vi "SR_Gen_Overview.vi"(11 "State Sample":refnum<class "RDS State.lvclass">) -> (2 "Overview":T1 {"Distance to Target" format="%.01f [meters]"; "Longitude" format="%.6g"; "Latitude" format="%.6g"; "Water Temp" format="%.0f [celcius]"; "Pitch" scale=45.0..-45.0; "Roll" scale=-20.0..20.0; "Current" format="%02.2f [amps]"; "Voltage" format="%02.2f [volts]"; "Capacity" format="%_1f [Percent]"; "Water Depth" format="%.01f [meters]"; "GPS Speed" format="%.01f [knots]"; "Compass" scale=0.36..360.0}, 3 "State Sample Out":refnum<class "RDS State.lvclass">)   [LabVIEW 2015, in "Shore Library.lvlib"]
uses:
  Shore Library.lvlib
  SR_Overview.ctl
  RDS State Tracker/RDS State/RDS State.lvclass
  RDS State Tracker/RDS State/RDS State.lvclass/RDS State.ctl
panel:
  # "Batteries"
  # "Actual Heading"
  # "Desired Heading"
  # "Throttle"
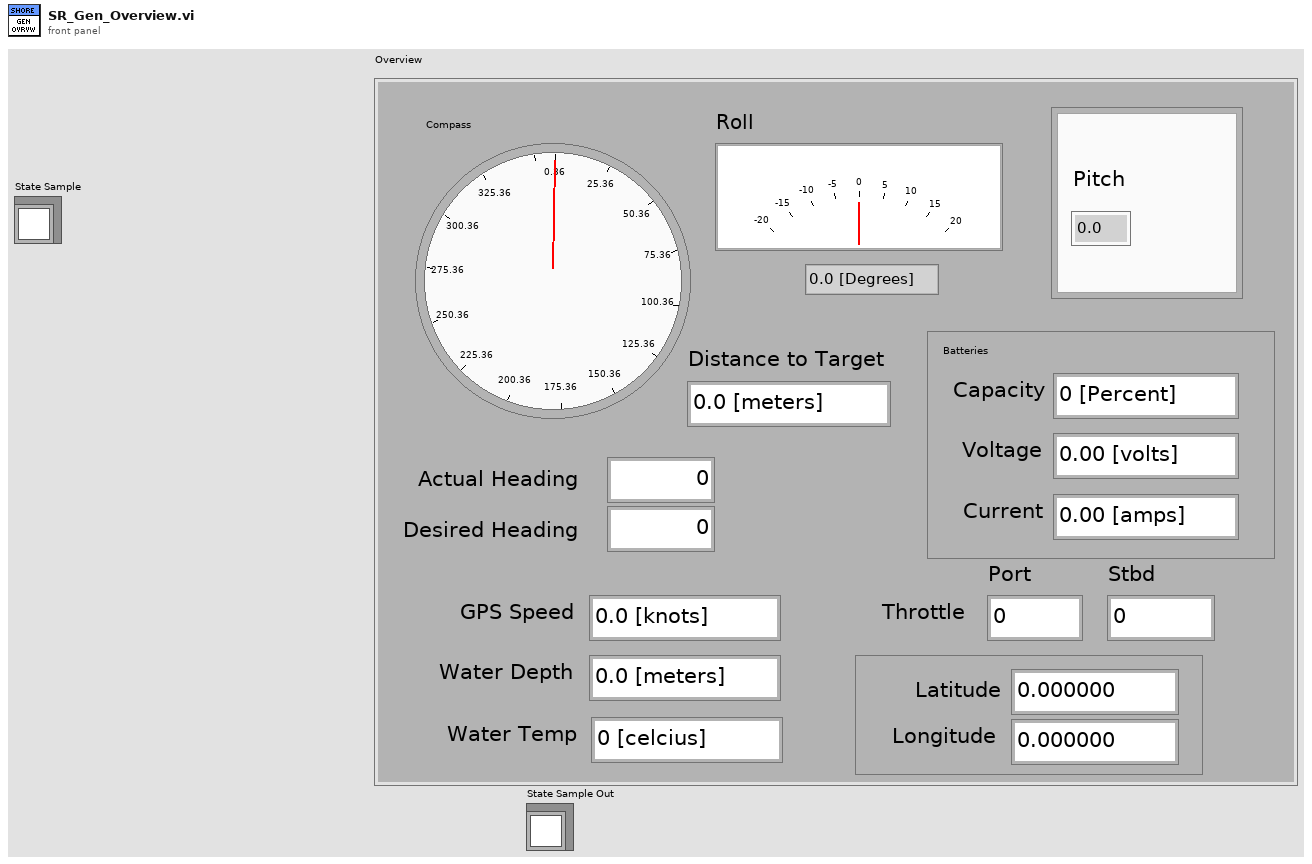
[diagram p1: front panel]
types:
  T1 = typedef "Shore Library.lvlib/SR_Overview.ctl" = cluster{"Throttle Stbd":dbl, "Compass":cluster{sgl, sgl}, "GPS Speed":dbl, "Water Depth":dbl, "Capacity":dbl, "Voltage":dbl, "Current":dbl, "Throttle Port":dbl, "Roll":sgl, "Pitch":sgl, "Water Temp":dbl, "Latitude":dbl, "Longitude":dbl, "Distance to Target":dbl}
  T2 = typedef "RDS Instrument Library.lvlib/Battery Data.ctl" = cluster{"Battery Status":T3, "Pack Voltage":sgl, "Pack Current":sgl, "Pack Capacity":sgl, "Max Cell Temp":sgl, "Min Cell Temp":sgl, "Max Cell Voltage":sgl, "Min Cell Voltage":sgl}
  T3 = typedef "RDS Instrument Library.lvlib/Battery Status.ctl" = enum16{"Pack Normal", "Alarm: Cell temp too high", "Alarm: Pack voltage too high", "Warn: Pack voltage too high ", "Alarm: Pack voltage too low", "Warn: Pack voltage low", "Alarm Pack current too high", "Warn: Pack current too high ", "Fault: Pack to chassis connection detected", "Fault: Pack to cell connection error", "Fautl: System error"}
  T4 = typedef "RDS Child Messages.lvlib/Depth Data.ctl" = cluster{"Depth":sgl, "Water Temp":i8}
  T5 = typedef "RDS Child Messages.lvlib/Helm Status Control.ctl" = cluster{"Helm State":T6, "Heading Command Control":T7, "Steering Command Control":T8, "Last Command Time":timestamp, "Gains":T9, "Current Heading":dbl, "Port Throttle":i16, "STBD Throttle":i16, "Limiter":dbl}
  T6 = typedef "RDS Helm Actor.lvlib/Helm State.ctl" = enum16{"Idle", "Executing Heading Command", "Executing Steering Command"}
  T7 = typedef "RDS Child Messages.lvlib/Heading Command Cntrl.ctl" = cluster{"Throttle":i16, "Heading":sgl, "Duration (s)":i16}
  T8 = typedef "RDS Child Messages.lvlib/Steering Command Cntrl.ctl" = cluster{"Throttle":i16, "Rudder":i8, "Duration (s)":u16}
  T9 = typedef "RDS Child Messages.lvlib/PID Gains Control.ctl" = cluster{"P (Kc)":sgl, "I (Ti)":sgl, "D (Td)":sgl}
  T10 = typedef "RDS Child Messages.lvlib/MCB Motor Status.ctl" = cluster{"Motor Power":i16, "Motor Command":i16, "Battery Volts":sgl, "Battery Amps":sgl, "Motor Amps":sgl, "MCU Temp":i16, "Heatsink Temp":i16, "Fault Flags":u16, "StatusFlags":u16}
  T11 = typedef "RDS Instrument Library.lvlib/Compass Data.ctl" = cluster{"Compass Heading":sgl, "pitch Angle":sgl, "roll Angle":sgl, "Temperature":sgl, "Depth":sgl, "Magnetic Field":sgl, "Magnetic Field X":sgl, "Magnetic Field Y":sgl, "Magnetic Field Z":sgl, "Acceleration":sgl, "Acceleration X":sgl, "Acceleration Y":sgl, "Gyro":sgl, "Gyro X":sgl, "Acceleration Z":sgl, "Gyro Y":sgl, "Raw Heading":sgl}
  T12 = typedef "RDS Libraries.lvlib/NMEA.lvlib/NMEA_GPRMC-data.ctl" = cluster{"TimeStamp":timestamp, "Validity":bool, "Latitude":dbl, "Latitude-Direction":T13, "Longitude":dbl, "Longitude-Direction":T14, "Speed in knots":sgl, "True course":sgl, "Date Stamp":timestamp, "Magnetic Variation (East/West)":sgl, "GPS Latitude":dbl, "GPS Longitude":dbl}
  T13 = typedef "RDS Libraries.lvlib/NMEA.lvlib/NMEA_LatitudeDirection.ctl" = enum16{"", "North", "South"}
  T14 = typedef "RDS Libraries.lvlib/NMEA.lvlib/NMEA_LongitudeDirection.ctl" = enum16{"", "East", "West"}
  T15 = typedef "RDS Child Messages.lvlib/Mission Controller State Message.lvclass/Mission Controller State Control.ctl" = cluster{"iHasControl":bool, "controlTimer":timestamp, "Nav State":T16, "Current MissionOp Index":i32, "Mission":T17[], "Distance to Target":dbl, "Seconds to Timeout":dbl}
  T16 = typedef "RDS Mission Controller Actor.lvlib/Mission Controller Navigation State.ctl" = cluster{"GPS Latitude":ext, "GPS Longitude":ext, "Compass Heading":dbl, "Speed":dbl}
  T17 = typedef "RDS Mission Controller Actor.lvlib/MissionOp.ctl" = cluster{"MissionOp Type":enum16{"Waypoint", "Loiter", "Wait", "Deploy AIP", "Stow AIP"}, "Duration (s)":u16, "Throttle":i16, "GPS Latitude":dbl, "GPS Longitude":dbl, "Loiter Range (m)":u16}
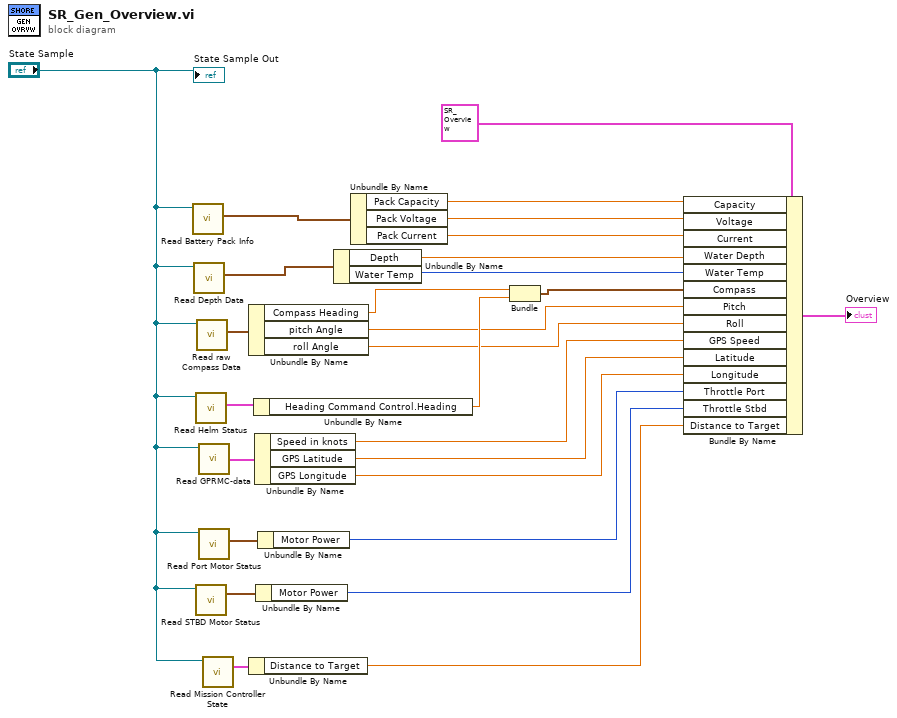
[diagram p0: block diagram]
diagram:
  n1 = call "Read Battery Pack Info.vi"("RDS State in"="State Sample") -> ("Battery Pack Info"=w27:T2)  [unwired: 8 in, 2 out]
  n2 = call "Read Depth Data.vi"("RDS State in"="State Sample") -> ("Depth Data"=w22:T4)  [unwired: 8 in, 2 out]
  n3 = call "Read Helm Status.vi"("RDS State in"="State Sample") -> ("Helm Status"=w19:T5)  [unwired: 8 in, 2 out]
  n4 = call "Read STBD Motor Status.vi"("RDS State in"="State Sample") -> ("STBD Motor"=w6:T10)  [unwired: 8 in, 2 out]
  n5 = call "Read raw Compass Data.vi"("RDS State in"="State Sample") -> ("Compass Data"=w18:T11)  [unwired: 8 in, 2 out]
  n6 = call "Read GPRMC-data.vi"("RDS State in"="State Sample") -> ("GPRMC-data"=w12:T12)  [unwired: 8 in, 2 out]
  n7 = call "Read Port Motor Status.vi"("RDS State in"="State Sample") -> ("Port Motor Data"=w8:T10)  [unwired: 8 in, 2 out]
  n8 = call "Read Mission Controller State.vi"("RDS State in"="State Sample") -> ("Mission Controller State"=w3:T15)  [unwired: 8 in, 2 out]
  n9 = Unbundle By Name(w18) -> ("Compass Heading"=w17:sgl, "pitch Angle"=w14:sgl, "roll Angle"=w13:sgl)
  n10 = Unbundle By Name(w3) -> ("Distance to Target"=w1:dbl)
  n11 = Unbundle By Name(w19) -> ("Heading Command Control.Heading"=w16:sgl)
  n12 = Unbundle By Name(w12) -> ("Speed in knots"=w11:sgl, "GPS Latitude"=w10:dbl, "GPS Longitude"=w9:dbl)
  n13 = Unbundle By Name(w6) -> ("Motor Power"=w5:i16)
  n14 = Unbundle By Name(w8) -> ("Motor Power"=w7:i16)
  n15 = Unbundle By Name(w22) -> ("Depth"=w21:sgl, "Water Temp"=w20:i8)
  n16 = Unbundle By Name(w27) -> ("Pack Capacity"=w26:sgl, "Pack Voltage"=w25:sgl, "Pack Current"=w24:sgl)
  n17 = Bundle("Compass Heading"=w17, "Heading"=w16) -> (w15:cluster{"Compass Heading":sgl, "Heading":sgl})  [unwired: 1 in]
  n18 = Bundle By Name(cluster=T1 {"Throttle Stbd"=0.0, "Compass"={7.9180083, 358.98358}, "GPS Speed"=0.0, "Water Depth"=0.0, "Capacity"=0.0, "Voltage"=0.0, "Current"=0.0, "Throttle Port"=0.0, "Roll"=6.186918, "Pitch"=-45.0, "Water Temp"=0.0, "Latitude"=0.0, "Longitude"=0.0, "Distance to Target"=0.0} ("Overview"), "Capacity"=w26, "Voltage"=w25, "Current"=w24, "Water Depth"=w21, "Water Temp"=w20, "Compass"=w15, "Pitch"=w14, "Roll"=w13, "GPS Speed"=w11, "Latitude"=w10, "Longitude"=w9, "Throttle Port"=w7, "Throttle Stbd"=w5, "Distance to Target"=w1) -> (→"Overview":T1)
  "State Sample Out" <- "State Sample"
